vi "Initialize.vi"(4 "Local(F)_Remote(T)":bool, 5 "Port":i32, 6 "Route(F)/Relay(T)":bool, 7 "Host IP":string, 8 "error in (no error)":errorcluster, 9 "Topology":string, 10 "Alias":string, 11 "Device/Resource Name":string) -> (0 "error out":errorcluster, 3 "SLSC Card Config out":refnum<class "SLSC Card Config.lvclass">)   [LabVIEW 2018, in "SLSC Card Config.lvclass"]
uses:
  Switch Configuration.llb/SLSC Card Config.lvclass
  C:/Users/jennifer.platt/Documents/Switch-Custom-Device - Copy/Source/Switch Card Config/Switch Card Config.lvclass
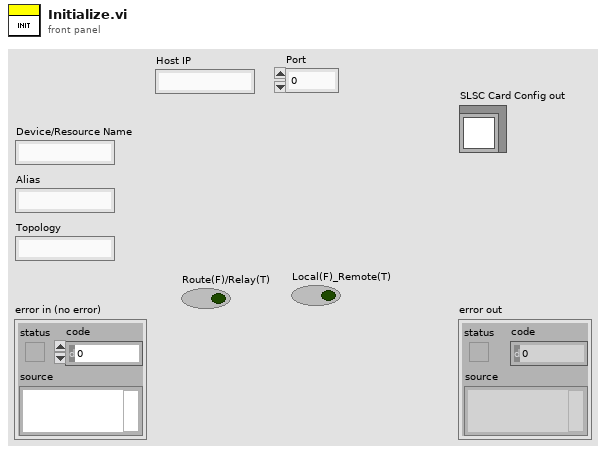
[diagram p1: front panel]
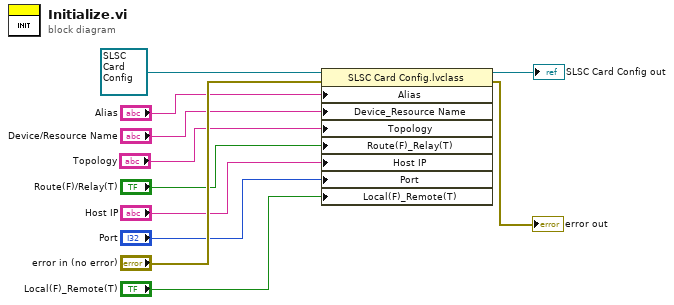
[diagram p0: block diagram]
diagram:
  n1 = property class="SLSC Card Config.lvclass"(reference=refnum<class "SLSC Card Config.lvclass"> refnum ("SLSC Card Config out"), error in="error in (no error)", "Alias"="Alias", "Device_Resource Name"="Device/Resource Name", "Topology"="Topology", "Route(F)_Relay(T)"="Route(F)/Relay(T)", "Host IP"="Host IP", "Port"="Port", "Local(F)_Remote(T)"="Local(F)_Remote(T)") -> (reference out=→"SLSC Card Config out":refnum<class "SLSC Card Config.lvclass">, error out=→"error out":errorcluster)
